vi "uv encode.vi"(8 "error in (no error)":errorcluster, 9 "para2":cluster{}, 10 "para1":dbl, 11 "para0":dbl) -> (0 "error out":errorcluster, 3 "function return":i32)   [LabVIEW 2018]
doc: "LIBTIFF_DLL_IMPEXP int uv_encode(double, double, int = SGILOGENCODE_NODITHER);"
uses:
  libtiff3.dll
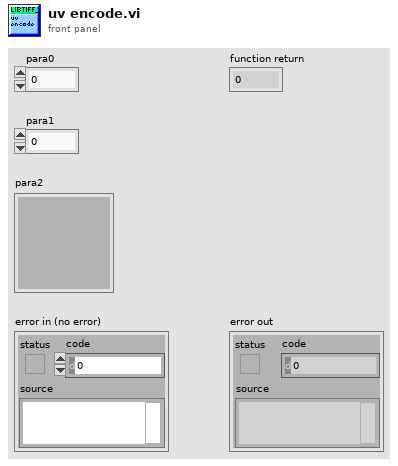
[diagram p1: front panel]
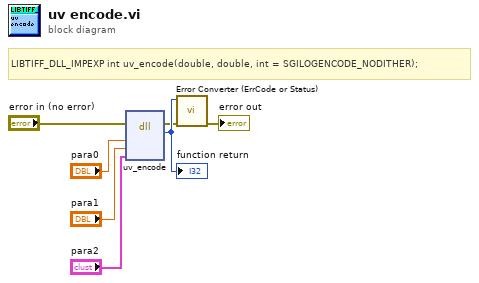
[diagram p0: block diagram]
diagram:
  # "LIBTIFF_DLL_IMPEXP\tint uv_encode(double, double, int = SGILOGENCODE_NODITHER);"
  n1 = dll-call lib="C:/Users/johan/Downloads/LabVIEW software/LabVIEW software/IX-81 Software/lib/tiff/LibTiffLabview/libtiff3.*" fn="uv_encode"(error in="error in (no error)", "para0"="para0", "para1"="para1", "para2"="para2") -> (error out=w2:errorcluster, w7:i32)  [unwired: 5 in, 1 out]
  "function return" <- w7
  n2 = call "Error Converter (ErrCode or Status).vi"("error in (no error)"=w2, "error code"=w7) -> ("error out"=→"error out":errorcluster)  [unwired: 9 in]
